vi "Generate Waveform.vi"() -> ()   [LabVIEW 2011, in "Dumb Plugin.lvclass"]
uses:
  Dumb Plugin.lvclass
  <vilib>/measure/NI_MABase.lvlib
panel:
  in  "Vertical Point Slide":dbl(slide) scale=0.0..10.0
  out "Waveform Graph":waveform(dbl)(graph)
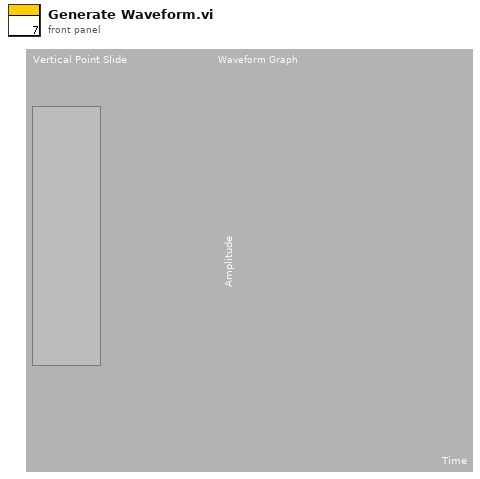
[diagram p1: front panel]
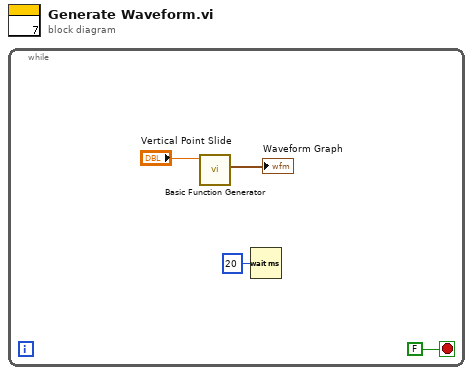
[diagram p0: block diagram]
diagram:
  n1 = while {
    stop <- FALSE stop-if-true
    n2 = call <vilib>:"Basic Function Generator.vi"("frequency"="Vertical Point Slide") -> ("signal out"=→"Waveform Graph":waveform(dbl))  [unwired: 8 in, 2 out]
    n3 = Wait (ms)(milliseconds to wait=u32 20) -> ()  [unwired: 1 out]
  }
